vi "get_resolution.vi"(8 "error in (no error)":errorcluster, 11 "TrajectoryMG100122AODFrameScan in":refnum<class "TrajectoryMG100122AODFrameScan.lvclass">) -> (0 "error out":errorcluster, 1 "y resolution":i32, 2 "x resolution":i32, 3 "TrajectoryMG100122AODFrameScan out":refnum<class "TrajectoryMG100122AODFrameScan.lvclass">)   [LabVIEW 2010, in "TrajectoryMG100122AODFrameScan.lvclass"]
uses:
  TrajectoryMG100122AODFrameScan.lvclass
  TrajectoryMG100122AODFrameScan.lvclass/TrajectoryMG100122AODFrameScan.ctl
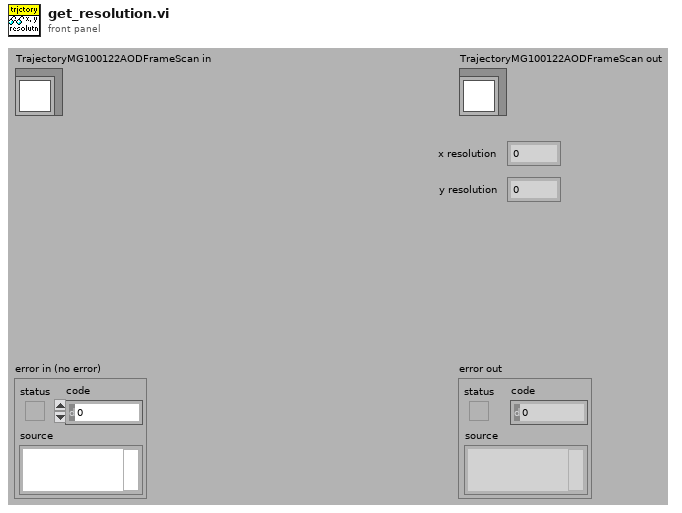
[diagram p1: front panel]
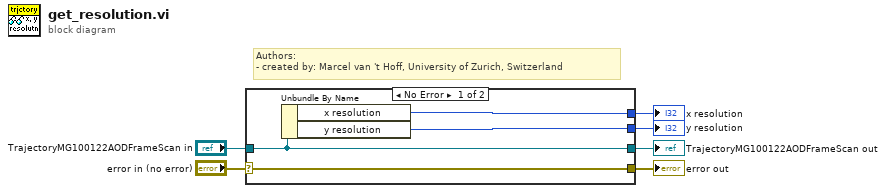
[diagram p0: block diagram]
diagram:
  # "Authors: \n- created by: Marcel van 't Hoff, University of Zurich, Switzerland"
  n1 = case shown="No Error" "error in (no error)" {
    selector: "error in (no error)" -> [w10 w11]
    tunnel: [w10 w11] -> w5
    tunnel: [w9 w12] -> w3
    tunnel: "TrajectoryMG100122AODFrameScan in" -> [w9 w12]
    tunnel: [w8 _] -> w2
    tunnel: [w7 _] -> w1
    frame No Error {
      n2 = Unbundle By Name(w9) -> ("x resolution"=w8:i32, "y resolution"=w7:i32)
    }
    frame Error {
    }
  }
  "error out" <- w5
  "TrajectoryMG100122AODFrameScan out" <- w3
  "x resolution" <- w2
  "y resolution" <- w1
